vi "Camera-GetImage.vi"(4 "Streeam":bool, 5 "Image Device IN":cluster{"Image":T1, "errorImage":errorcluster}, 8 "Camera Device IN":T2) -> (0 "Image Device OUT":cluster{"Image":T1, "errorImage":errorcluster}, 3 "Camera Device OUT":T2)   [LabVIEW 2010]
uses:
  <vilib>/vision/Image Controls.llb/IMAQ Image.ctl
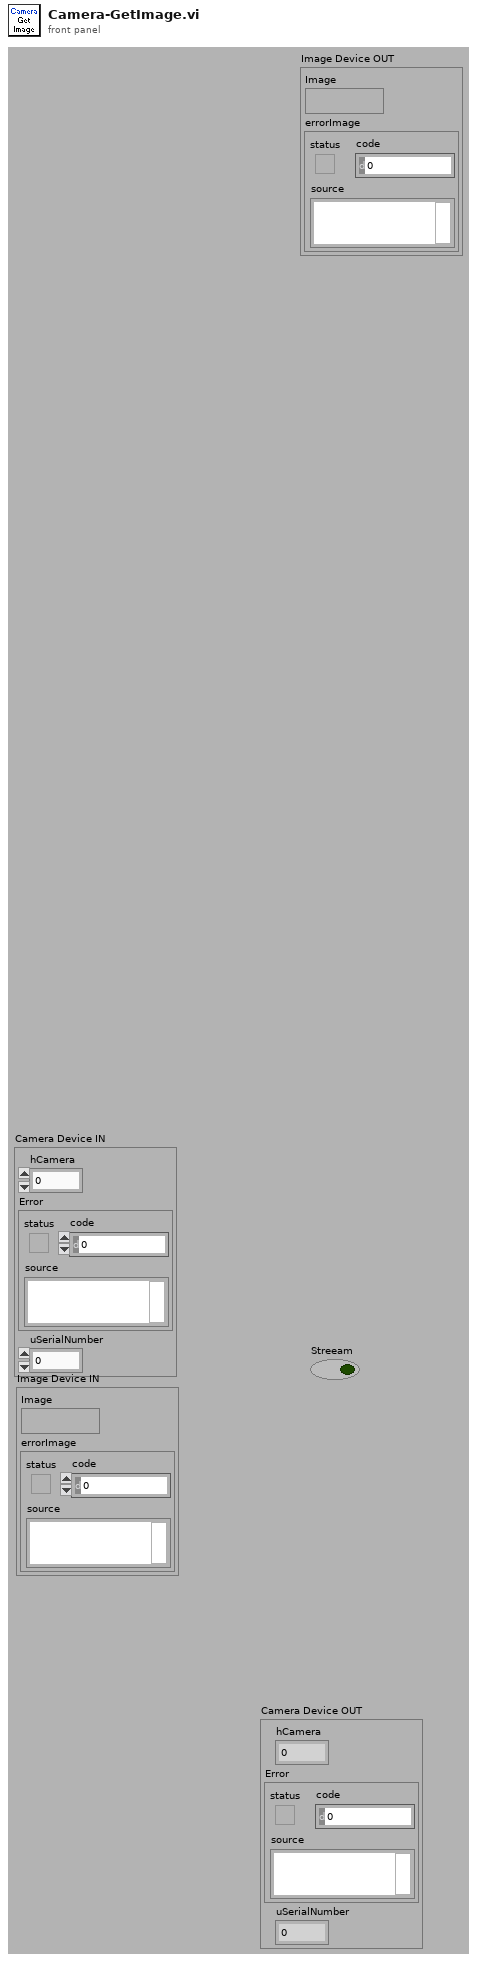
[diagram p1: front panel]
types:
  T1 = typedef "IMAQ Image.ctl" = refnum<image>
  T2 = cluster{"hCamera":u32, "Error":errorcluster, "uSerialNumber":u32}
  T3 = enum32{"Map Pixel Pointer", "Unmap Pixel Pointer", "Get Pixels Infos"}
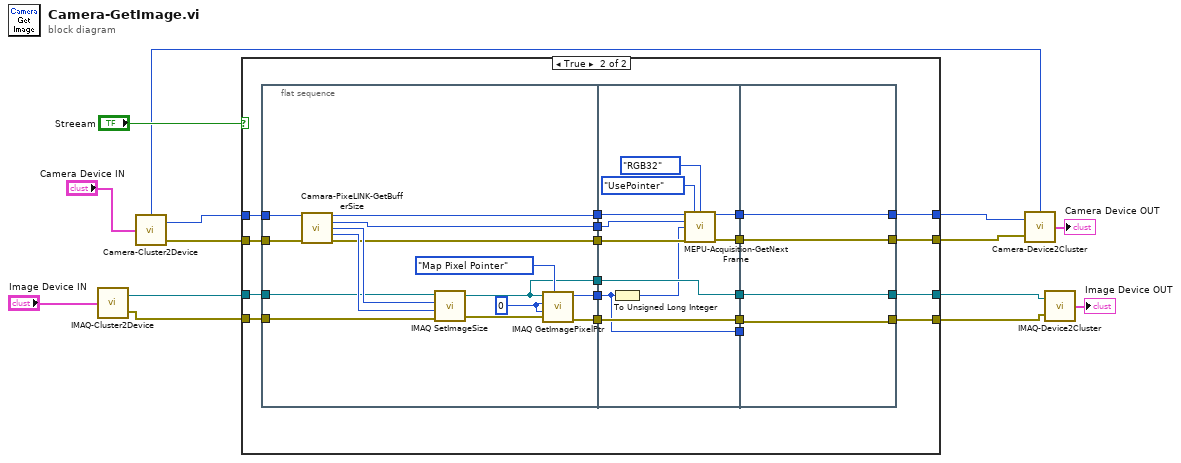
[diagram p0: block diagram]
diagram:
  n1 = call "IMAQ-Cluster2Device.vi"("Image Device IN"="Image Device IN") -> ("errorImage OUT"=w2:errorcluster, "Image OUT"=w3:T1)
  n2 = call "Camera-Cluster2Device.vi"("Camera Device IN"="Camera Device IN") -> ("Error OUT"=w9:errorcluster, "hCamera OUT"=w10:u32, "uSerialNumber OUT"=w7:u32)  [unwired: 2 in]
  n3 = case shown="True" "Streeam" {
    tunnel: w10 -> [w18 w32]
    tunnel: w9 -> [w17 w31]
    tunnel: w3 -> [w16 w30]
    tunnel: w2 -> [w15 w29]
    tunnel: [w16 w28] -> w5
    tunnel: [w15 w27] -> w4
    tunnel: [w17 w26] -> w12
    tunnel: [w18 w25] -> w13
    frame False {
    }
    frame True {
      n4 = flat-sequence {
        tunnel: [w38] -> w37
        tunnel: [w39] -> w36
        tunnel: w30 -> [w50]
        tunnel: w29 -> [w49]
        tunnel: w32 -> [w48]
        tunnel: w31 -> [w47]
        tunnel: [w44] -> w35
        tunnel: [w43] -> w34
        tunnel: [w42] -> w33
        tunnel: [w41] -> w24
        tunnel: w37 -> [w63]
        tunnel: w36 -> [w62]
        tunnel: w35 -> [w53]
        tunnel: w34 -> [w56]
        tunnel: w33 -> [w57]
        tunnel: w24 -> [w61]
        tunnel: [w58] -> w23
        tunnel: [w57] -> w22
        tunnel: [w56] -> w21
        tunnel: [w55] -> w20
        tunnel: [w53] -> w19
        tunnel: [w66] -> w26
        tunnel: [w64] -> w27
        tunnel: [w65] -> w28
        tunnel: [w67] -> w25
        tunnel: w23 -> [w67]
        tunnel: w22 -> [w65]
        tunnel: w21 -> [w64]
        tunnel: w20 -> [w66]
        tunnel: w19 -> [_]
        frame #0 {
          w40 = 0 ("Y Coordinate")
          n5 = call "Camara-PixeLINK-GetBufferSize.vi"("phCamera IN"=w48, "Error IN"=w47) -> ("phCamera OUT"=w38:u32, "uBufferSize OUT"=w41:u32, "uWidth OUT"=w52:u32, "uHeight OUT"=w51:u32, "Error OUT"=w39:errorcluster)  [unwired: 9 out]
          n6 = call "IMAQ SetImageSize"("error in (no error)"=w49, "Y Resolution"=w51, "X Resolution"=w52, "Image"=w50) -> ("error out"=w46:errorcluster, "Image Out"=w42:T1)  [unwired: 1 in]
          n7 = call "IMAQ GetImagePixelPtr"("Function"=T3."Map Pixel Pointer", "error in (no error)"=w46, "Y Coordinate"=w40, "X Coordinate"=w40, "Image"=w42) -> ("error out"=w43:errorcluster, "Pixel Pointer out"=w44:u64)  [unwired: 1 in, 4 out]
        }
        frame #1 {
          n8 = To Unsigned Long Integer(number=w53) -> (unsigned 32bit integer=w54:u32)
          n9 = call <vilib>:"MEPU-Acquisition-GetNextFrame.vi"("hCamera IN"=w63, "Mode IN"=enum16{"UseArray", "UsePointer"}."UsePointer", "OutputMode IN"=enum16{"Default", "RGB24", "RGB32"}."RGB32", "uBufferSize IN"=w61, "pPixel IN"=w54, "Error IN"=w62) -> ("hCamera OUT"=w58:u32, "Error OUT"=w55:errorcluster)  [unwired: 5 in, 3 out]
        }
        frame #2 {
        }
      }
    }
  }
  n10 = call "Camera-Device2Cluster.vi"("uSerialNumber IN"=w7, "Error IN"=w12, "hCamera IN"=w13) -> ("Camera Device OUT"=→"Camera Device OUT":T2)
  n11 = call "IMAQ-Device2Cluster.vi"("errorImage IN"=w4, "Image IN"=w5) -> ("Image Device OUT"=→"Image Device OUT":cluster{"Image":T1, "errorImage":errorcluster})
